vi "Read Error Counts.vi"(8 "error in":errorcluster, 11 "Rx execution unit in":refnum<class "Rx Execution Unit.lvclass">) -> (0 "error out":errorcluster, 2 "error counts":T1, 3 "Rx execution unit out":refnum<class "Rx Execution Unit.lvclass">)   [LabVIEW 2020, in "AIM ARINC 429 Engine.lvlib" / "Implementation.lvlib" / "Rx Execution Unit.lvclass"]
uses:
  Rx Execution Unit.lvclass
  Rx Execution Unit.lvclass/Rx Execution Unit.ctl
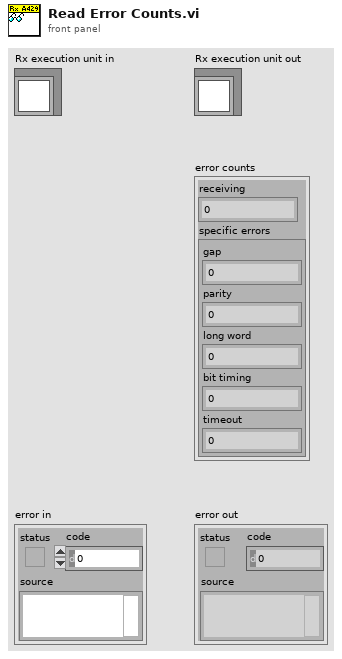
[diagram p1: front panel]
types:
  T1 = cluster{"receiving":dbl, "specific errors":cluster{"gap":dbl, "parity":dbl, "long word ":dbl, "bit timing":dbl, "timeout":dbl}}
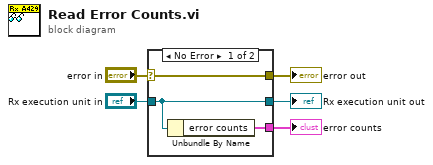
[diagram p0: block diagram]
diagram:
  n1 = case shown="No Error" "error in" {
    selector: "error in" -> [w8 w9]
    tunnel: [w8 w9] -> w4
    tunnel: [w7 w10] -> w2
    tunnel: "Rx execution unit in" -> [w7 w10]
    tunnel: [w6 _] -> w1
    frame No Error {
      n2 = Unbundle By Name(w7) -> ("error counts"=w6:T1)
    }
    frame Error {
    }
  }
  "error out" <- w4
  "Rx execution unit out" <- w2
  "error counts" <- w1
